vi "Abort Fit Global.vi"() -> ()   [LabVIEW 2019]
panel:
  out "Abort Fit":bool
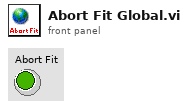
[diagram p1: front panel]
diagram:
